vi "ScanBarcode.vi"(10 "VISA引用句柄输入":refnum<visa-resource-name>) -> (0 "TimeOut":bool, 2 "HodlerID":string, 3 "BarcodeData":string)   [LabVIEW 2017]
panel:
  out "Left":bool
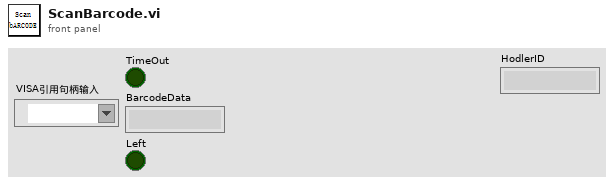
[diagram p1: front panel]
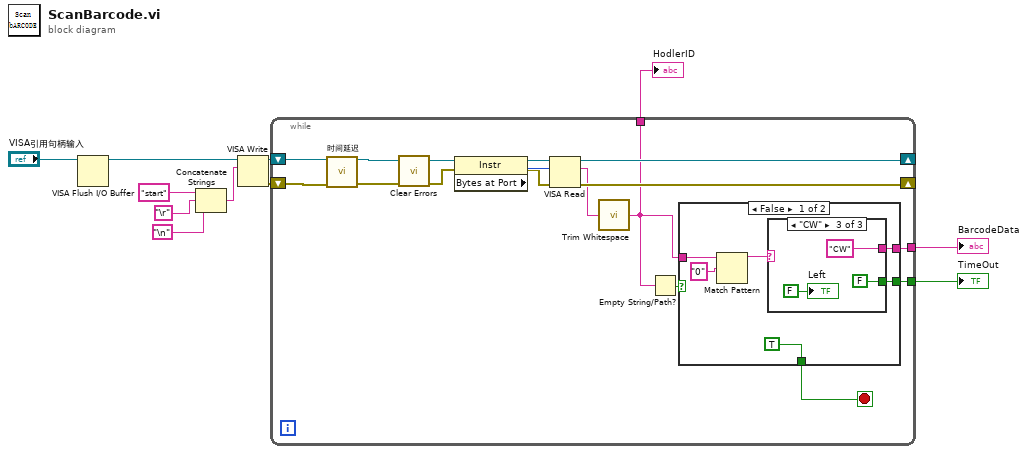
[diagram p0: block diagram]
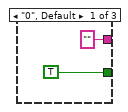
[diagram p2: hidden frame]
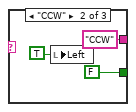
[diagram p3: hidden frame]
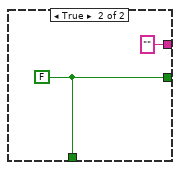
[diagram p4: hidden frame]
diagram:
  n1 = VISA Flush I/O Buffer(VISA resource name="VISA引用句柄输入") -> (VISA resource name out=w1:refnum<visa-resource-name>)  [unwired: 2 in, 1 out]
  n2 = Concatenate Strings("start" ("write buffer"), "\r", "\n") -> (w9:string)
  n3 = VISA Write(VISA resource name=w1, write buffer=w9) -> (VISA resource name out=w10:refnum<visa-resource-name>, error out=w11:errorcluster)  [unwired: 1 in, 1 out]
  n4 = while {
    shift-right: [w20] -> _
    shift-left: w11 -> [w22]
    shift-right: [w19] -> _
    shift-left: w10 -> [w23]
    tunnel: [w15] -> w5
    tunnel: [w14] -> w4
    tunnel: [w13] -> w2
    stop <- w16 stop-if-true
    n5 = call "时间延迟"("error in (no error)"=w22) -> ("error out"=w12:errorcluster)  [unwired: 10 in]
    n6 = call <vilib>:"Clear Errors.vi"("error in (no error)"=w12) -> ("error out"=w21:errorcluster)  [unwired: 5 in, 1 out]
    n7 = property class="Instr"(reference=w23, error in=w21) -> (reference out=w26:refnum<visa-resource-name>, error out=w24:errorcluster, "Bytes at Port"=w25:u32)
    n8 = VISA Read(VISA resource name=w26, byte count=w25, error in (no error)=w24) -> (VISA resource name out=w19:refnum<visa-resource-name>, read buffer=w17:string, error out=w20:errorcluster)  [unwired: 1 out]
    n9 = call <vilib>:"Trim Whitespace.vi"("string"=w17) -> ("trimmed string"=w13:string)  [unwired: 1 in]
    n10 = Empty String/Path?(string/path=w13) -> (empty?=w18:bool)
    n11 = case shown="False" w18 {
      tunnel: w13 -> [w28 _]
      tunnel: [TRUE w42] -> w16
      tunnel: [w30 w42] -> w15
      tunnel: [w29 ""] -> w14
      frame False {
        n12 = Match Pattern(string=w28, regular expression="0") -> (before substring=w27:string)  [unwired: 1 in, 3 out]
        n13 = case shown="\"CW\"" w27 {
          tunnel: [TRUE FALSE FALSE] -> w30
          tunnel: ["" "CCW" "CW"] -> w29
          frame "0", Default {
          }
          frame "CCW" {
            n14 = local write "Left"(TRUE) -> ()
          }
          frame "CW" {
            "Left" <- FALSE
          }
        }
      }
      frame True {
        w42 = FALSE
      }
    }
  }
  "TimeOut" <- w5
  "BarcodeData" <- w4
  "HodlerID" <- w2
